vi "Version Update.vi"(8 "error in (no error)":errorcluster, 10 "Version":cluster{i32, i32, i32}, 11 "Device Item Ref In in":T1 format="%.0x") -> (0 "error out":errorcluster, 3 "Device Item Ref In out":T1 format="%.0x")   [LabVIEW 2017, in "PXImc System Explorer.lvlib"]
uses:
  PXImc System Explorer.lvlib
  <vilib>/NI Veristand/Custom Device API/Custom Device Item Ref.ctl
  Shared/Constants.vi
  <vilib>/NI VeriStand/Custom Device API/Custom Device API.lvlib
  Shared/PXImc Shared.lvlib
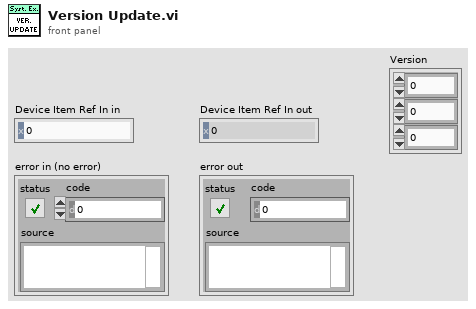
[diagram p1: front panel]
types:
  T1 = typedef "Custom Device API.lvlib/Custom Device Item Ref.ctl" = u64
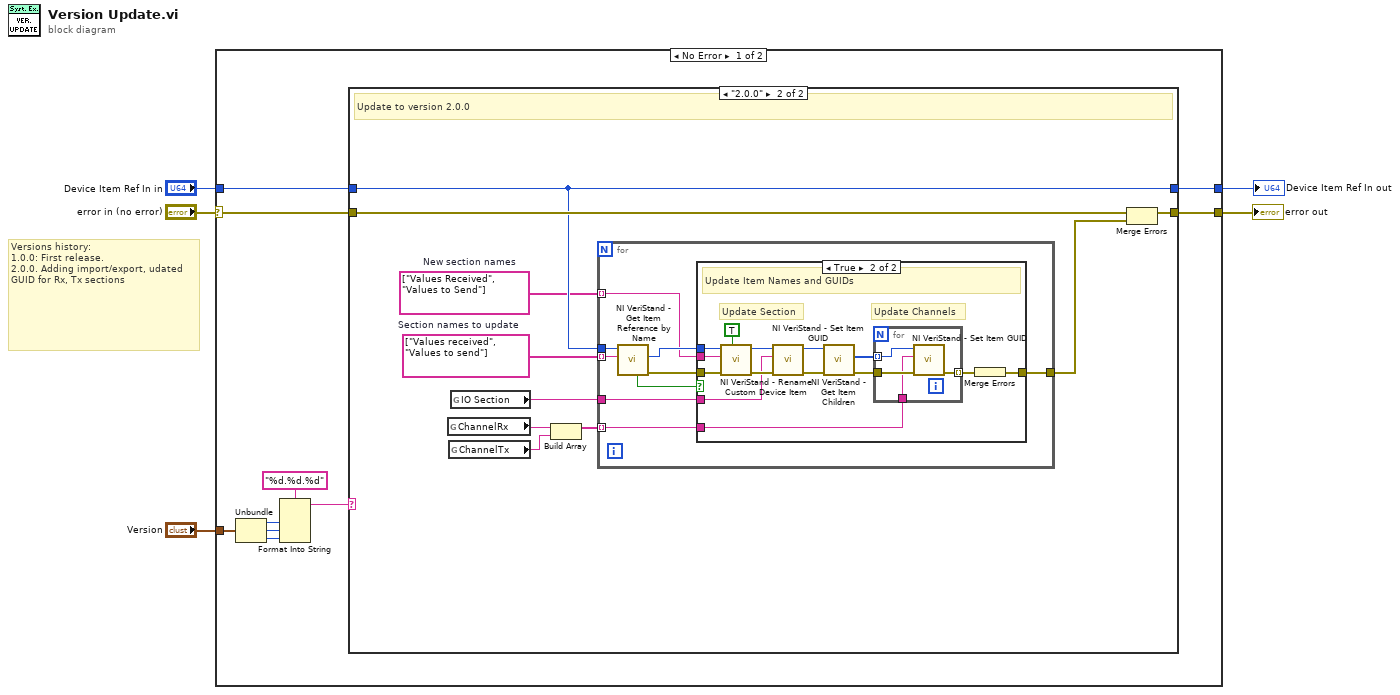
[diagram p0: block diagram]
diagram:
  # "Versions history:\n1.0.0: First release.\n2.0.0. Adding import/export, udated GUID for Rx, Tx sections"
  n1 = case shown="No Error" "error in (no error)" {
    selector: "error in (no error)" -> [w13 w56]
    tunnel: "Device Item Ref In in" -> [w14 w57]
    tunnel: [w15 w57] -> w3
    tunnel: [w12 w56] -> w2
    tunnel: "Version" -> [w11 _]
    frame No Error {
      n2 = Unbundle(w11) -> (w10:i32, w9:i32, w8:i32)
      n3 = Format Into String(format string="%d.%d.%d", w10, w9, w8) -> (resulting string=w6:string)  [unwired: 2 in, 1 out]
      n4 = case shown="\"2.0.0\"" w6 {
        tunnel: [w17 w19] -> w15
        tunnel: w14 -> [w17 w19]
        tunnel: w13 -> [w16 w26]
        tunnel: [w16 w27] -> w12
        frame Default {
        }
        frame "2.0.0" {
          w18 = string[] ["Values Received", "Values to Send"]  # New section names
          w23 = string[] ["Values received", "Values to send"]  # Section names to update
          # "Update to version 2.0.0"
          n5 = global read "Constants.vi" "ChannelRx"() -> (w21:string)
          n6 = global read "Constants.vi" "ChannelTx"() -> (w20:string)
          n7 = global read "Constants.vi" "IO Section"() -> (w24:string)
          n8 = Build Array(w21, w20) -> (w22:string[])
          n9 = for {
            tunnel: w23 -> [w36] mode=indexing
            tunnel: w19 -> [w35]
            tunnel: [w31] -> w25
            tunnel: w24 -> [w30]
            tunnel: w22 -> [w29] mode=indexing
            tunnel: w18 -> [w28] mode=indexing
            n10 = call <vilib>:"NI VeriStand - Get Item Reference by Name.vi"("Item Name"=w36, "Parent Ref in"=w35) -> ("error out"=w32:errorcluster, "Item Ref"=w33:T1, "Found"=w34:bool)  [unwired: 6 in, 1 out]
            n11 = case shown="True" w34 {
              tunnel: w33 -> [_ w50]
              tunnel: w32 -> [w37 w51]
              tunnel: [w37 w41] -> w31
              tunnel: w30 -> [_ w40]
              tunnel: w29 -> [_ w39]
              tunnel: w28 -> [_ w38]
              frame False {
              }
              frame True {
                # "Update Channels"
                # "Update Section"
                # "Update Item Names and GUIDs"
                n12 = call <vilib>:"NI VeriStand - Rename Custom Device Item.vi"("Force Rename (F)"=TRUE, "error in (no error)"=w51, "New Name"=w38, "Item Ref in"=w50) -> ("error out"=w48:errorcluster, "Item Ref out"=w47:T1)  [unwired: 5 in, 1 out]
                n13 = call <vilib>:"NI VeriStand - Set Item GUID.vi"("error in (no error)"=w48, "GUID"=w40, "Item Ref in"=w47) -> ("error out"=w45:errorcluster, "Item Ref out"=w46:T1)  [unwired: 7 in]
                n14 = call <vilib>:"NI VeriStand - Get Item Children.vi"("error in (no error)"=w45, "Item Ref in"=w46) -> ("error out"=w43:errorcluster, "Child Refs"=w44:T1[])  [unwired: 6 in, 2 out]
                n15 = for {
                  tunnel: w44 -> [w55] mode=indexing
                  tunnel: w43 -> [w54]
                  tunnel: [w53] -> w42 mode=indexing
                  tunnel: w39 -> [w52]
                  n16 = call <vilib>:"NI VeriStand - Set Item GUID.vi"("error in (no error)"=w54, "GUID"=w52, "Item Ref in"=w55) -> ("error out"=w53:errorcluster)  [unwired: 7 in, 1 out]
                }
                n17 = Merge Errors(w42) -> (w41:errorcluster)
              }
            }
          }
          n18 = Merge Errors(w26, w25) -> (w27:errorcluster)
        }
      }
    }
    frame Error {
    }
  }
  "error out" <- w2
  "Device Item Ref In out" <- w3
